vi "Main.vi"() -> ()   [LabVIEW 2015]
doc: "This template is for the Queued Message Handler design pattern.\n\nThe Event Handling Loop generates messages based on user interface actions.\n\nThe Message Handling Loop processes messages generated by the Event Handling Loop, or by other messages. The messages are string values, so new messages can be added easily to the Message Cases case structure in the Message Handling Loop. Each message cluster can also provide an optional value for Message Data, which is a variant that can be converted to whatever message-specific data is required."
uses:
  controls/Instruments.ctl
  controls/UI Data.ctl
  controls/UI Config.ctl
  Classes/Calibrator.lvclass
  Classes/34410A.lvclass
  Classes/34401A.lvclass
  Classes/8846A.lvclass
  Classes/8845A.lvclass
  Classes/U1252.lvclass
  Classes/U1213A.lvclass
  Classes/189.lvclass
  Classes/289/289.lvclass
  Classes/TY720.lvclass
  Classes/Multimeter.lvclass
  controls/Ini File Output.ctl
  support/Message Queue/Enqueue Message (Single).vi
  <vilib>/Utility/config.llb/Read Key (String).vi
  support/Developer VIs/Write Cell.vi
  support/Developer VIs/Write Cell String.vi
  <vilib>/Utility/error.llb/Error Cluster From Error Code.vi
  <vilib>/Utility/NIReport.llb/NI_report.lvclass
  <vilib>/ErrorRing/Error Ring.xnode
  support/Message Queue/Message Queue.lvlib
  support/User Event - Stop/User Event - Stop.lvlib
  <vilib>/Utility/config.llb/NI_LVConfig.lvlib
  <vilib>/addons/_office/NI_ReportGenerationToolkit.lvlib
panel:
  out "Conexão com Padrão":bool
  in  "Frequência":bool=TRUE
  in  "Bobina":enum16{"50", "75"}(ring)
  in  "Capacitância":bool=TRUE
  in  "Próxima Calibração":timestamp format="%<%x>T"
  in  "Multimetro":T1
  in  "Corrente AC":bool=TRUE
  in  "Corrente DC":bool=TRUE
  in  "Parar":bool
  in  "Número de Controle":string
  in  "Patrimônio":string
  in  "Tipo de Calibração":enum32{"Nova", "Recalibração"}(radio)
  in  "Tensão DC":bool=TRUE
  in  "Tensão AC":bool=TRUE
  in  "Resistência":bool=TRUE
  in  "Finalizar Aplicativo":bool
  in  "Iniciar Calibração":bool
  # "CALIBRAÇÃO AUTOMÁTICA\nDE MULTÍMETROS DIGITAIS"
  # "Selecione as Grandezas\nElétricas"
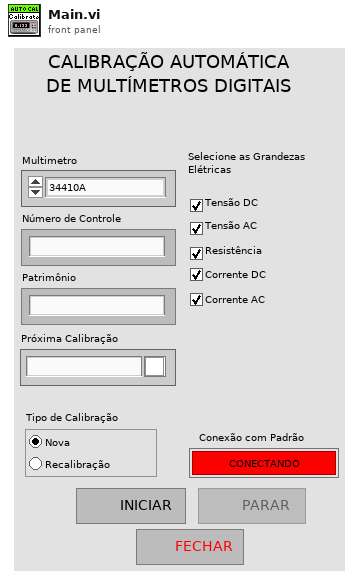
[diagram p1: front panel]
types:
  T1 = typedef "Instruments.ctl" = enum16{"34410A", "34401A", "U1252B", "U1252A", "U1213A", "8845A", "8846A", "189", "289", "DMM4050", "TY720"}
  T2 = typedef "UI Data.ctl" = cluster{"Voltage DC":refnum<vi>, "Voltage AC":refnum<vi>, "Resistance":refnum<vi>, "Current DC":refnum<vi>, "Current AC":refnum<vi>, "Finalizar":refnum<vi>, "Iniciar Cal":refnum<vi>, "Stop":refnum<vi>, "Conexão com Padrão":refnum<vi>, "Número de Controle":refnum<vi>, "Patrimônio":refnum<vi>, "Próxima Calibração":refnum<vi>, "Tipo de Calibração":refnum<vi>, "Bobina":refnum<vi>, "Capacitância":refnum<vi>, "Frequência":refnum<vi>, "Bobina":refnum<vi>, "Multimetro":refnum<vi>}
  T3 = typedef "Message Queue.lvlib/All Message Queues.ctl" = cluster{"UI":refnum<queue>}
  T4 = typedef "UI Config.ctl" = enum16{"Initial Config", "Calibration Config"}
  T5 = enum16{"Standard Report", "HTML", "Word", "Excel"}
  T6 = enum16{"maximized", "minimized", "normal", "no change"}
  T7 = typedef "NI_LVConfig.lvlib/Config Data RefNum.ctl" = refnum<k1>
  T8 = typedef "Ini File Output.ctl" = cluster{"Grandeza":string, "Cel Inicio":string, "Cel Fim":string, "Frequencia":dbl, "Delay":dbl, "Valor":dbl, "Num Medições":i32, "Cel Write":string, "Multiplicador":dbl, "Message":string, "Escala":dbl, "Reset":bool}
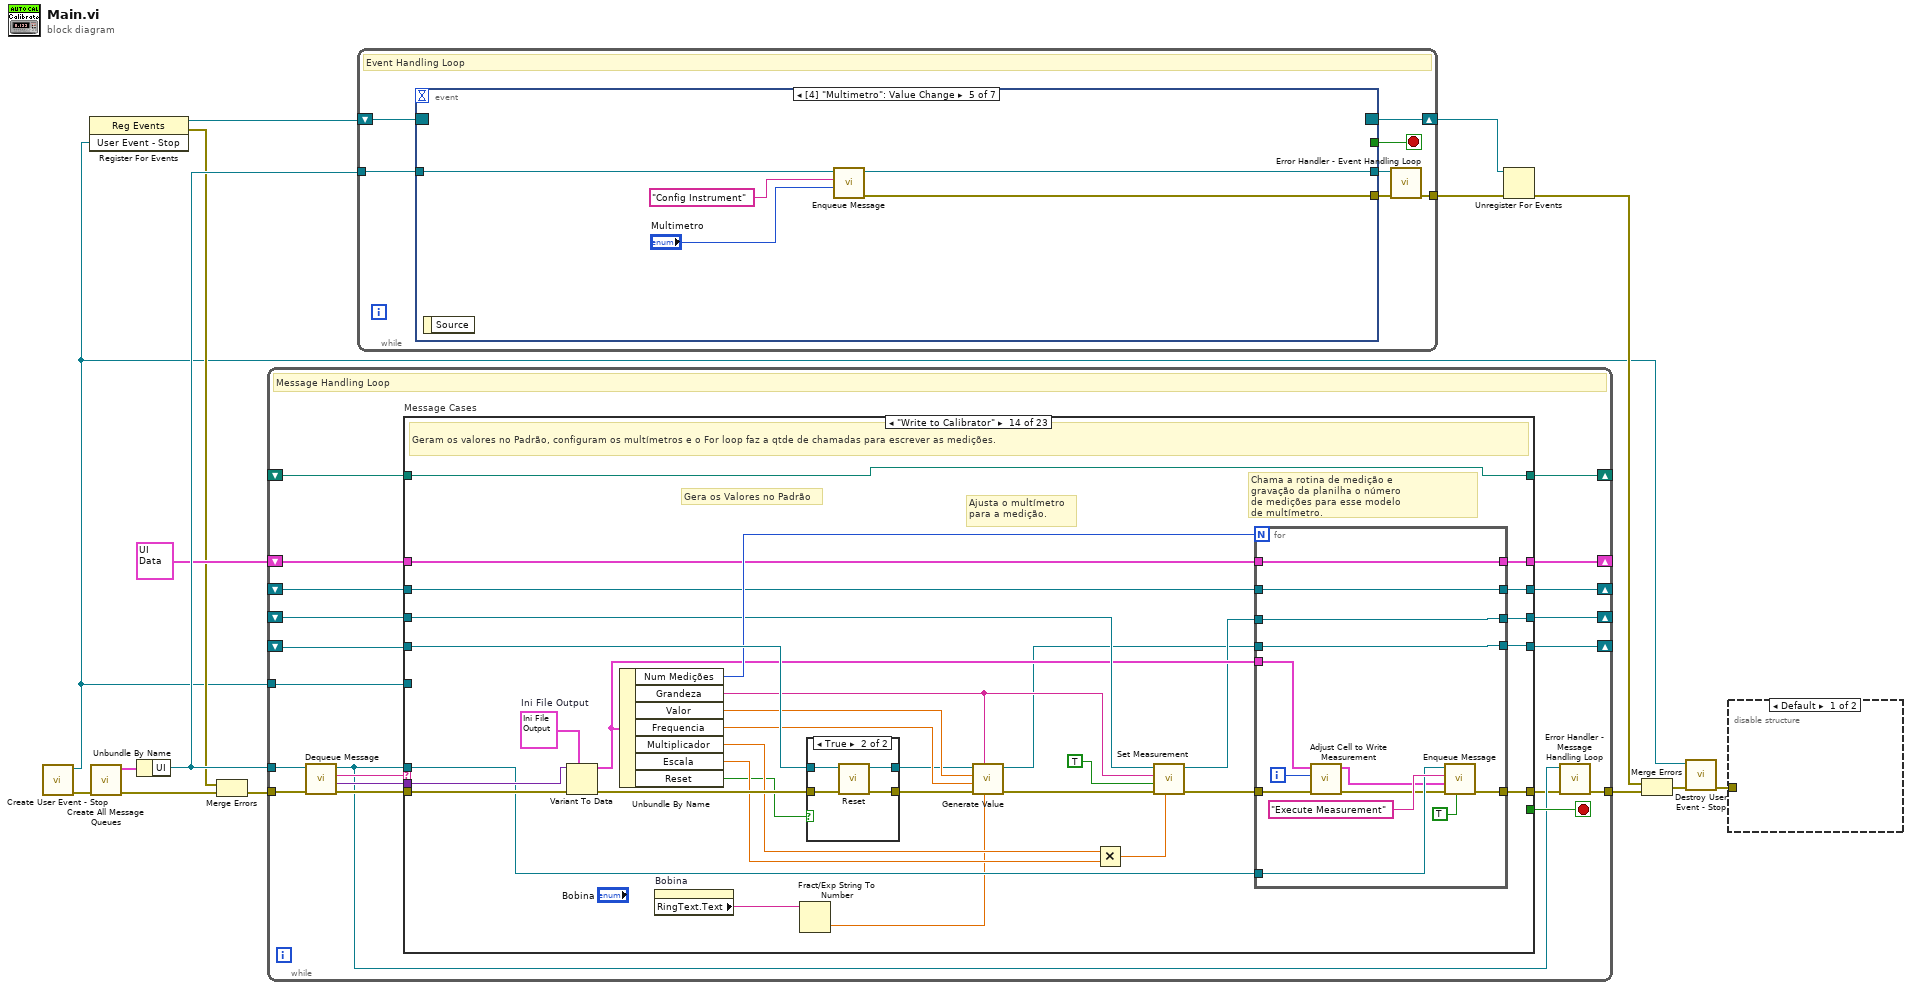
[diagram p0: block diagram]
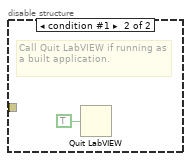
[diagram p2: hidden frame]
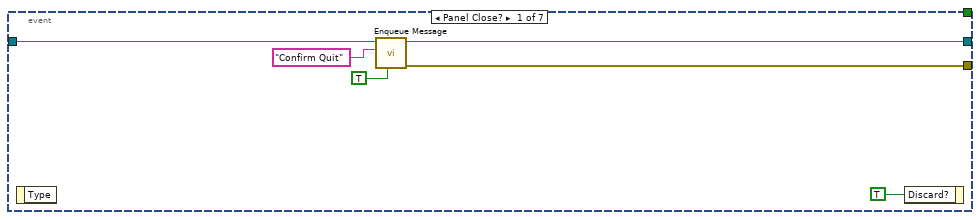
[diagram p3: hidden frame]
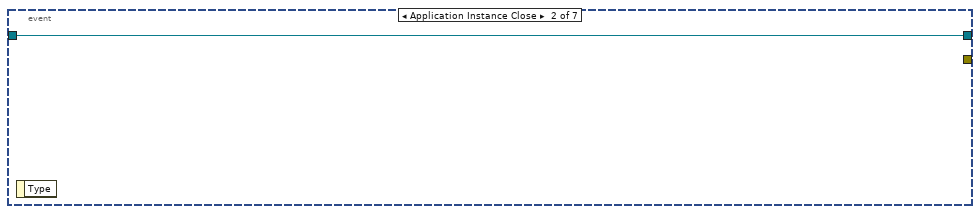
[diagram p4: hidden frame]
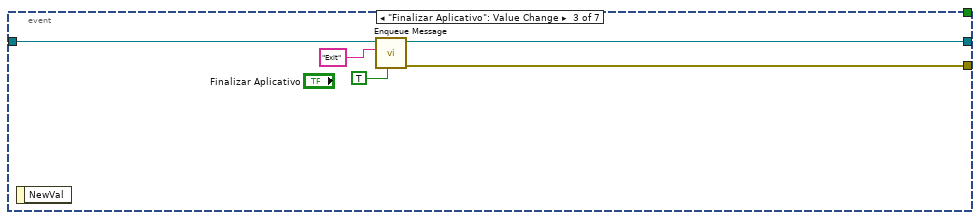
[diagram p5: hidden frame]
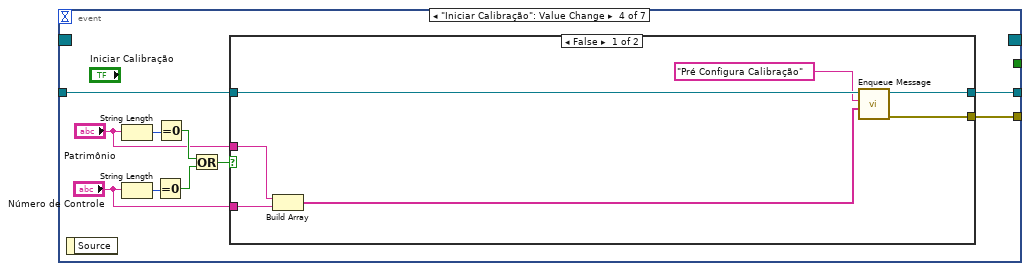
[diagram p6: hidden frame]
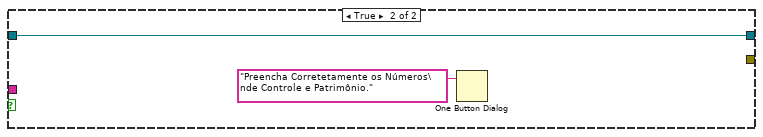
[diagram p7: hidden frame]
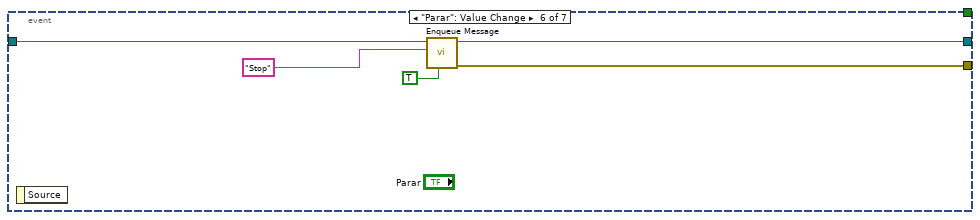
[diagram p8: hidden frame]
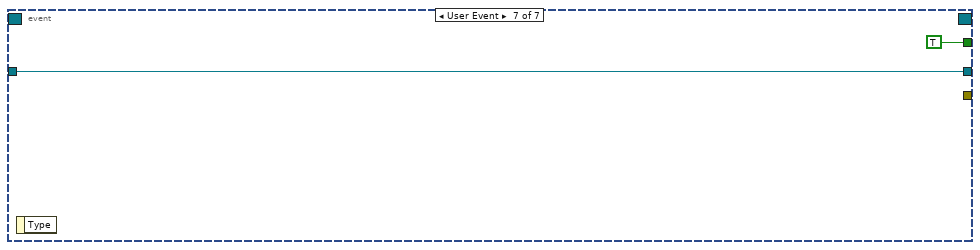
[diagram p9: hidden frame]
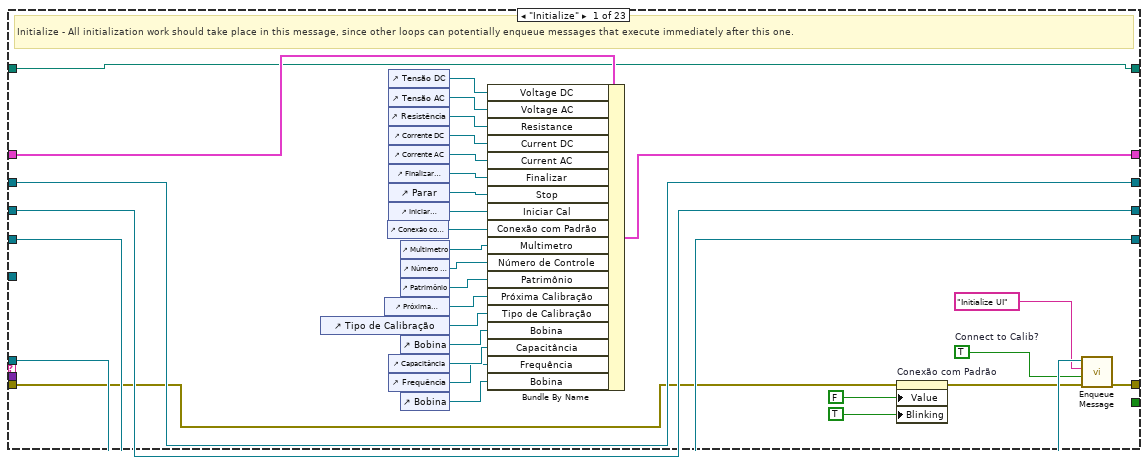
[diagram p10: hidden frame]
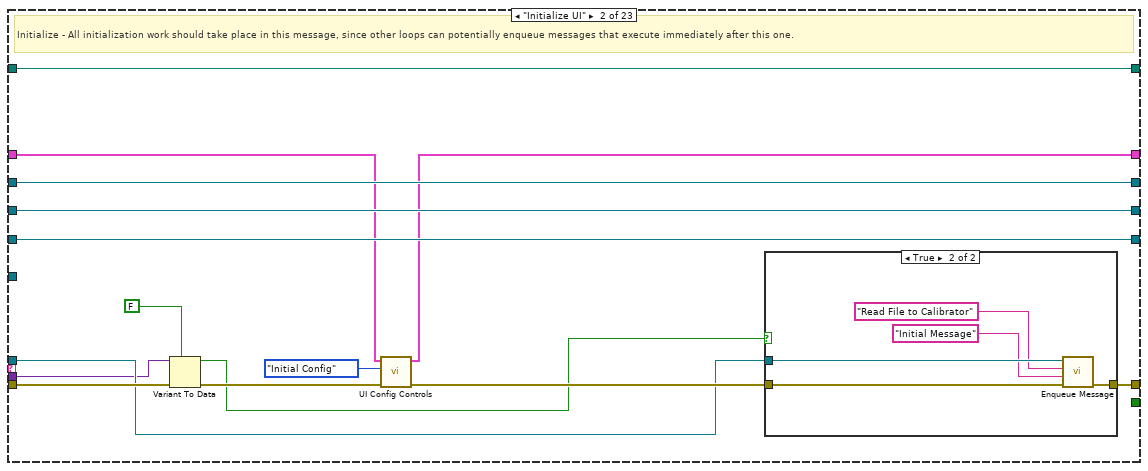
[diagram p11: hidden frame]
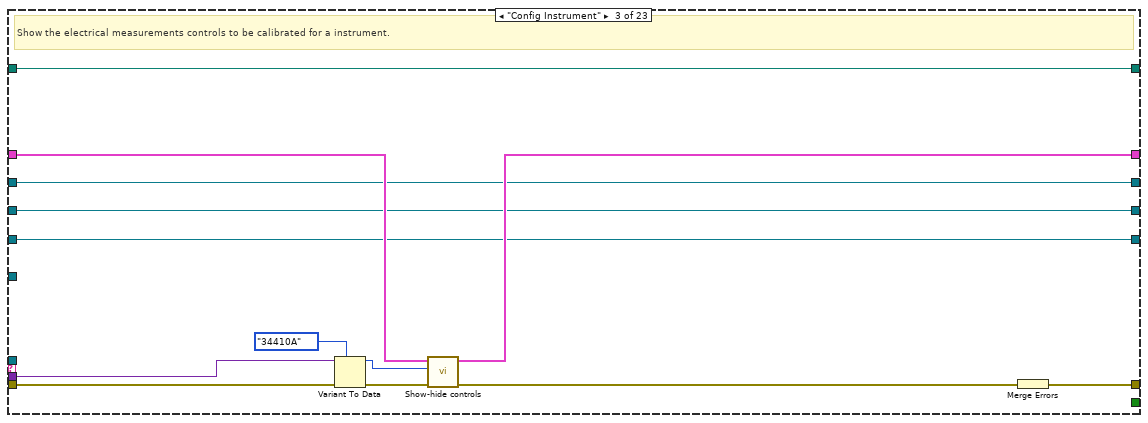
[diagram p13: hidden frame]
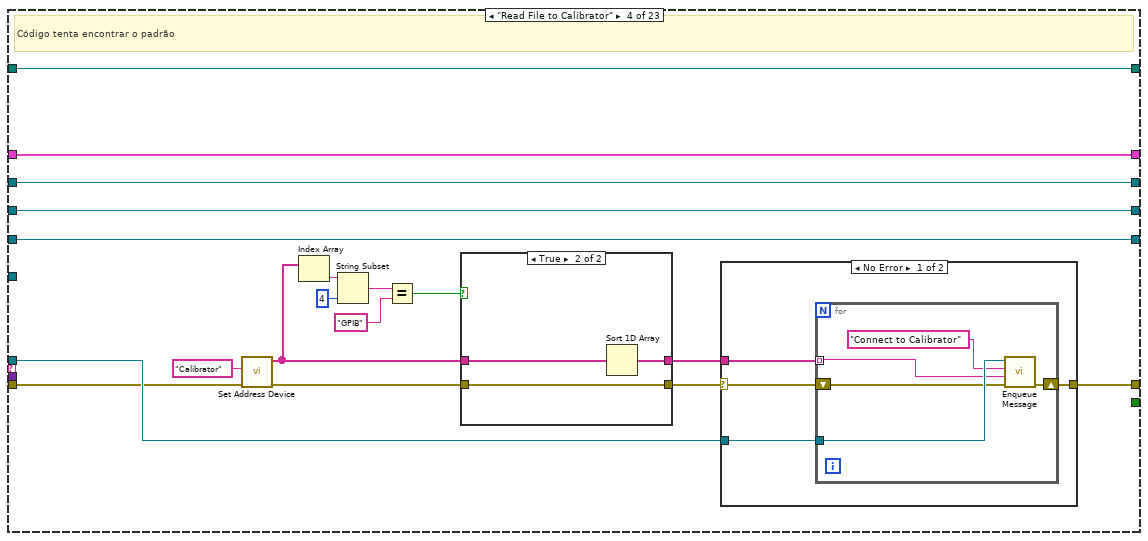
[diagram p14: hidden frame]
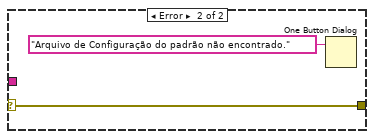
[diagram p16: hidden frame]
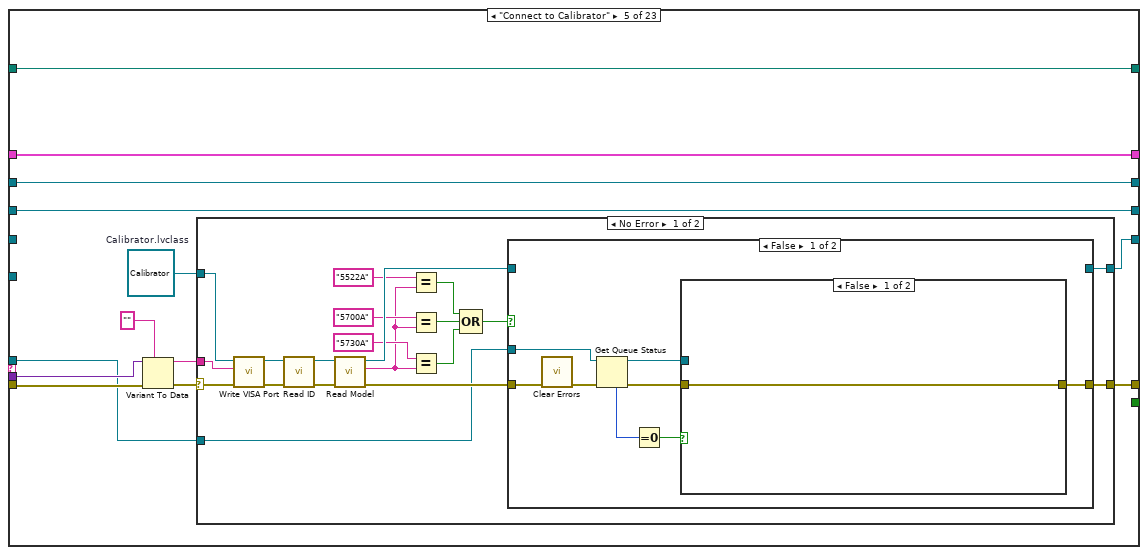
[diagram p17: hidden frame]
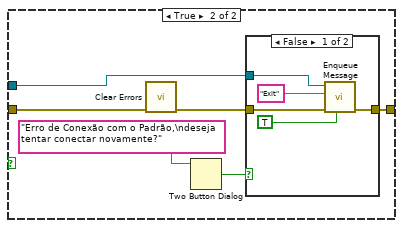
[diagram p18: hidden frame]
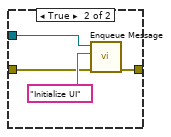
[diagram p19: hidden frame]
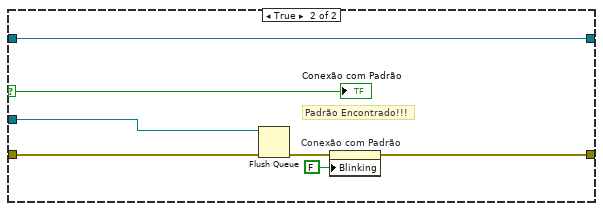
[diagram p20: hidden frame]
diagram:
  n1 = call "Create User Event - Stop.vi"() -> ("error out"=w11:errorcluster, "User Event - Stop"=w1:refnum<user-event>)  [unwired: 10 in]
  n2 = register-events(w1) -> (reference out=w4:refnum<event-registration>, error out=w2:errorcluster)  [unwired: 2 in]
  n3 = call "Create All Message Queues.vi"("error in (no error)"=w11) -> ("error out"=w15:errorcluster, "Message Queues out"=w14:T3)  [unwired: 9 in]
  n4 = Unbundle By Name(w14) -> ("UI"=w12:refnum<queue>)
  n5 = Merge Errors(w2, w15) -> (w3:errorcluster)
  n6 = while {
    tunnel: w12 -> [w27]
    shift-right: [w34] -> _
    shift-left: T2 {"Voltage DC"=refnum, "Voltage AC"=refnum, "Resistance"=refnum, "Current DC"=refnum, "Current AC"=refnum, "Finalizar"=refnum, "Iniciar Cal"=refnum, "Stop"=refnum, "Conexão com Padrão"=refnum, "Número de Controle"=refnum, "Patrimônio"=refnum, "Próxima Calibração"=refnum, "Tipo de Calibração"=refnum, "Bobina"=refnum, "Capacitância"=refnum, "Frequência"=refnum, "Bobina"=refnum, "Multimetro"=refnum} ("Data Cluster") -> [w35]
    tunnel: w1 -> [w32]
    tunnel: w3 -> [w31]
    tunnel: [w25] -> w13
    shift-right: [w18] -> _
    shift-left: _ -> [w23]
    shift-right: [w22] -> _
    shift-left: _ -> [w21]
    shift-right: [w20] -> _
    shift-left: _ -> [w19]
    shift-right: [w17] -> _
    shift-left: _ -> [w16]
    stop <- w33 stop-if-true
    # "Message Handling Loop"
    n7 = call "Dequeue Message.vi"("error in (no error)"=w31, "Message Queue"=w27) -> ("error out"=w30:errorcluster, "Message Data"=w28:variant, "Message"=w29:string, "dup Message Queue"=w26:refnum<queue>)  [unwired: 6 in]
    n8 = case "Message Cases" shown="\"Write to Calibrator\"" w29 {
      selector: w29 -> [_ _ _ _ _ _ _ _ _ _ _ _ _ _ _ _ _ _ _ _ _ _ w892]
      tunnel: w26 -> [w66 w73 _ w117 w138 w204 w246 w283 w356 _ w480 w529 _ w675 w718 w747 _ w841 w850 _ _ w887 _]
      tunnel: w30 -> [w40 w78 w98 w114 w143 w210 w245 w292 w352 w464 w490 w546 w618 w684 w728 w753 w806 w840 w854 w861 w868 w882 _]
      tunnel: [w67 w82 w101 w118 w136 w205 w241 w284 w339 w443 w476 w539 w614 w674 w714 w744 w800 w809 w852 w859 w867 w885 w893] -> w24
      tunnel: w35 -> [w65 w77 w95 w119 w148 w214 w240 w291 w363 w468 w492 w545 w605 w656 w729 w737 w805 w808 w853 w860 w866 w878 w894]
      tunnel: [w59 w76 w93 w119 w148 w214 w239 w291 w363 w468 w492 w545 w606 w655 w729 w736 w805 w807 w853 w860 w866 w876 w894] -> w34
      tunnel: [_ _ _ _ _ _ _ _ _ _ _ _ _ _ _ _ _ _ _ _ _ TRUE _] -> w33
      tunnel: w28 -> [_ w69 w100 _ w141 _ w244 w290 w351 w463 w489 w538 w613 w683 w727 w752 w804 _ _ _ _ w879 _]
      tunnel: w32 -> [_ _ _ _ _ _ _ _ _ _ _ _ _ _ _ _ _ _ _ _ _ w884 _]
      tunnel: [w53 w81 w92 w112 w137 w207 w258 w282 w362 w467 w491 w534 w609 w658 w723 w739 w799 w813 w847 w858 w865 w871 w891] -> w18
      tunnel: w23 -> [w53 w81 w92 w112 _ w208 w258 w289 w362 w467 w491 w535 w610 w680 w723 w740 w799 w815 w847 w858 w865 w872 w891]
      tunnel: [w56 w80 w91 w116 w147 w213 w257 w280 w342 w466 w472 w543 w616 w662 w721 w745 w798 w818 w846 w857 w864 w875 w890] -> w22
      tunnel: w21 -> [w56 w80 w91 w116 w147 w213 w257 _ w343 w466 w473 w544 w617 w671 w722 w746 w798 w818 w846 w857 w864 w875 w890]
      tunnel: [w46 w79 w90 w115 w146 w212 w256 w276 w346 w459 w482 w537 w612 w660 w712 w750 w797 w820 w845 w856 w863 w874 w889] -> w20
      tunnel: w19 -> [w46 w79 w90 w115 w146 w212 w256 w276 w346 w459 w482 w536 w611 w661 w724 _ w797 w834 w845 w856 w863 w874 w889]
      tunnel: [w42 w72 w89 w113 w145 w201 w230 w272 w338 w441 w469 w528 w604 w654 w704 w735 w796 w819 w844 w855 w862 w869 w888] -> w17
      tunnel: w16 -> [w42 w72 w89 w113 w145 w201 w230 w272 w338 w441 w469 w528 w604 w654 w704 _ w796 w819 w844 w855 w862 w869 w888]
      frame "Initialize" {
        w41 = TRUE  # Connect to Calib?
        # "Initialize - All initialization work should take place in this message, since other loops can potentially enqueue messages that execute immediately after this one."
        n9 = control-ref of="Tipo de Calibração"() -> (w51:refnum<vi>)
        n10 = control-ref of="Próxima Calibração"() -> (w50:refnum<vi>)
        n11 = control-ref of="Conexão com Padrão"() -> (w39:refnum<vi>)
        n12 = control-ref of="Tensão DC"() -> (w64:refnum<vi>)
        n13 = control-ref of="Tensão AC"() -> (w63:refnum<vi>)
        n14 = control-ref of="Resistência"() -> (w62:refnum<vi>)
        n15 = control-ref of="Corrente DC"() -> (w61:refnum<vi>)
        n16 = control-ref of="Corrente AC"() -> (w60:refnum<vi>)
        n17 = control-ref of="Finalizar Aplicativo"() -> (w58:refnum<vi>)
        n18 = control-ref of="Parar"() -> (w55:refnum<vi>)
        n19 = control-ref of="Iniciar Calibração"() -> (w57:refnum<vi>)
        n20 = control-ref of="Capacitância"() -> (w47:refnum<vi>)
        n21 = control-ref of="Frequência"() -> (w45:refnum<vi>)
        n22 = control-ref of="Multimetro"() -> (w43:refnum<vi>)
        n23 = control-ref of="Número de Controle"() -> (w48:refnum<vi>)
        n24 = control-ref of="Patrimônio"() -> (w49:refnum<vi>)
        n25 = control-ref of="Bobina"() -> (w52:refnum<vi>)
        n26 = control-ref of="Bobina"() -> (w44:refnum<vi>)
        n27 = Bundle By Name(cluster=w65, "Voltage DC"=w64, "Voltage AC"=w63, "Resistance"=w62, "Current DC"=w61, "Current AC"=w60, "Finalizar"=w58, "Stop"=w55, "Iniciar Cal"=w57, "Conexão com Padrão"=w39, "Multimetro"=w43, "Número de Controle"=w48, "Patrimônio"=w49, "Próxima Calibração"=w50, "Tipo de Calibração"=w51, "Bobina"=w52, "Capacitância"=w47, "Frequência"=w45, "Bobina"=w44) -> (w59:T2)
        n28 = property on="Conexão com Padrão" class="Bool (strict)"(error in=w40, "Value"=FALSE ("Blinking"), "Blinking"=TRUE) -> (error out=w38:errorcluster)  [unwired: 1 in, 1 out]
        n29 = call-poly "Enqueue Message.vi"("error in (no error)"=w38, "Message Data"=w41, "Message"="Initialize UI", "Message Queue"=w66) -> ("error out"=w67:errorcluster)  [unwired: 6 in, 1 out]
      }
      frame "Initialize UI" {
        # "Initialize - All initialization work should take place in this message, since other loops can potentially enqueue messages that execute immediately after this one."
        n30 = Variant To Data(error in=w78, type=FALSE, Variant=w69) -> (data=w68:bool, error out=w71:errorcluster)
        n31 = call "UI Config Controls.vi"("Error In"=w71, "UI Configuration"=UI_Config."Initial Config", "UI Data"=w77) -> ("Error Out"=w74:errorcluster, "UI Data 2"=w76:T2)  [unwired: 7 in]
        n32 = case shown="True" w68 {
          tunnel: [w83 w88] -> w82
          tunnel: w74 -> [w83 w87]
          tunnel: w73 -> [_ w86]
          frame False {
          }
          frame True {
            n33 = call-poly "Enqueue Message.vi"("error in (no error)"=w87, "Message Data"="Initial Message" ("Initial Message"), "Message"="Read File to Calibrator", "Message Queue"=w86) -> ("error out"=w88:errorcluster)  [unwired: 6 in, 1 out]
          }
        }
      }
      frame "Config Instrument" {
        # "Show the electrical measurements controls to be calibrated for a instrument."
        n34 = Variant To Data(error in=w98, type=Instruments."34410A" ("Multimetro"), Variant=w100) -> (data=w96:T1, error out=w97:errorcluster)
        n35 = call "Show-hide controls.vi"("Error In"=w97, "Multimetro"=w96, "Data In"=w95) -> ("Error Out"=w94:errorcluster, "Data Out"=w93:T2)  [unwired: 7 in]
        n36 = Merge Errors(w94) -> (w101:errorcluster)
      }
      frame "Read File to Calibrator" {
        # "Código tenta encontrar o padrão"
        n37 = call "Set Address Device.vi"("error in (no error)"=w114, "Device"="Calibrator") -> ("error out"=w103:errorcluster, "find list"=w104:string[])  [unwired: 8 in]
        n38 = Index Array(array=w104) -> (element=w109:string)  [unwired: 1 in]
        n39 = String Subset(string=w109, length (rest)=4 ("length (rest)")) -> (substring=w106:string)  [unwired: 1 in]
        n40 = Equal?(x=w106, y="GPIB") -> (x = y?=w107:bool)
        n41 = case shown="True" w107 {
          tunnel: [w120 w124] -> w111
          tunnel: w104 -> [w120 w123]
          tunnel: w103 -> [w121 w122]
          tunnel: [w121 w122] -> w102
          frame False {
          }
          frame True {
            n42 = Sort 1D Array(array=w123) -> (sorted array=w124:string[])
          }
        }
        n43 = case shown="No Error" w102 {
          selector: w102 -> [w126 w135]
          tunnel: [w128 w135] -> w118
          tunnel: w117 -> [w127 _]
          tunnel: w111 -> [w125 _]
          frame No Error {
            n44 = for {
              tunnel: w127 -> [w132]
              shift-right: [w133] -> w128
              shift-left: w126 -> [w131]
              tunnel: w125 -> [w130] mode=indexing
              n45 = call-poly "Enqueue Message.vi"("error in (no error)"=w131, "Message Data"=w130, "Message"="Connect to Calibrator", "Message Queue"=w132) -> ("error out"=w133:errorcluster)  [unwired: 6 in, 1 out]
            }
          }
          frame Error {
            n46 = One Button Dialog(message="Arquivo de Configuração do padrão não encontrado.") -> ()  [unwired: 1 in, 1 out]
          }
        }
      }
      frame "Connect to Calibrator" {
        w144 = refnum<class "Calibrator.lvclass"> refnum  # Calibrator.lvclass
        n47 = Variant To Data(error in=w143, type="", Variant=w141) -> (data=w140:string, error out=w139:errorcluster)
        n48 = case shown="No Error" w139 {
          selector: w139 -> [w160 w200]
          tunnel: w144 -> [w168 _]
          tunnel: [w165 w200] -> w136
          tunnel: w138 -> [w164 _]
          tunnel: [w163 _] -> w137
          tunnel: w140 -> [w161 _]
          frame No Error {
            n49 = call-dynamic "Write VISA Port.vi"("error in (no error)"=w160, "VISA Port"=w161, "Device in"=w168) -> ("error out"=w158:errorcluster, "Device out"=w159:refnum<class "Calibrator.lvclass">)  [unwired: 7 in]
            n50 = call-dynamic "Read ID.vi"("error in (no error)"=w158, "Calibrator in"=w159) -> ("error out"=w156:errorcluster, "Calibrator out"=w157:refnum<class "Calibrator.lvclass">)  [unwired: 8 in]
            n51 = call-dynamic "Read Model.vi"("error in (no error)"=w156, "Device in"=w157) -> ("error out"=w166:errorcluster, "Model"=w153:string, "Device out"=w162:refnum<class "Calibrator.lvclass">)  [unwired: 7 in]
            n52 = Equal?(x="5522A", y=w153) -> (x = y?=w151:bool)
            n53 = Equal?(x="5700A", y=w153) -> (x = y?=w150:bool)
            n54 = Equal?(x="5730A", y=w153) -> (x = y?=w149:bool)
            n55 = Compound Arithmetic op=OR(w151, w150, w149) -> (w167:bool)
            n56 = case shown="False" w167 {
              selector: w167 -> [_ w198]
              tunnel: w166 -> [w171 w194]
              tunnel: [w176 w197] -> w165
              tunnel: w164 -> [w175 w195]
              tunnel: [_ w196] -> w163
              tunnel: w162 -> [_ w196]
              frame False {
                n57 = call <vilib>:"Clear Errors.vi"("error in (no error)"=w171) -> ("error out"=w170:errorcluster)  [unwired: 5 in, 1 out]
                n58 = Get Queue Status(queue=w175, error in (no error)=w170) -> (queue out=w172:refnum<queue>, error out=w173:errorcluster, # elements in queue=w169:i32)  [unwired: 1 in, 5 out]
                n59 = Equal To 0?(x=w169) -> (x = 0?=w174:bool)
                n60 = case shown="False" w174 {
                  tunnel: [w177 w181] -> w176
                  tunnel: w172 -> [_ w180]
                  tunnel: w173 -> [w177 w179]
                  frame False {
                  }
                  frame True {
                    n61 = call <vilib>:"Clear Errors.vi"("error in (no error)"=w179) -> ("error out"=w178:errorcluster)  [unwired: 5 in, 1 out]
                    n62 = Two Button Dialog(message="Erro de Conexão com o Padrão,\ndeseja tentar conectar novamente?") -> (T button?=w182:bool)  [unwired: 2 in]
                    n63 = case shown="False" w182 {
                      tunnel: w178 -> [w186 w189]
                      tunnel: [w185 w191] -> w181
                      tunnel: w180 -> [w184 w190]
                      frame False {
                        n64 = call-poly "Enqueue Message.vi"("Priority Message? (F)"=TRUE, "error in (no error)"=w186, "Message"="Exit", "Message Queue"=w184) -> ("error out"=w185:errorcluster)  [unwired: 6 in, 1 out]
                      }
                      frame True {
                        n65 = call-poly "Enqueue Message.vi"("error in (no error)"=w189, "Message"="Initialize UI", "Message Queue"=w190) -> ("error out"=w191:errorcluster)  [unwired: 7 in, 1 out]
                      }
                    }
                  }
                }
              }
              frame True {
                # "Padrão Encontrado!!!"
                n66 = Flush Queue(queue=w195, error in (no error)=w194) -> (error out=w193:errorcluster)  [unwired: 2 out]
                n67 = property on="Conexão com Padrão" class="Bool (strict)"(error in=w193, "Blinking"=FALSE) -> (error out=w197:errorcluster)  [unwired: 1 in, 1 out]
                "Conexão com Padrão" <- w198
              }
            }
          }
          frame Error {
          }
        }
      }
      frame "Checa Padrão" {
        n68 = call "FGV Config File.vi"("Error In"=w210, "Set/Get"=enum16{"Get", "Set"}."Get") -> ("Error Out"=w209:errorcluster, "Padrão Out"=w202:string[])  [unwired: 7 in, 1 out]
        n69 = for {
          tunnel: w209 -> [w229]
          tunnel: w208 -> [w228]
          tunnel: [w227] -> w207
          tunnel: [w226] -> w203
          tunnel: [w224] -> w206
          tunnel: w202 -> [w223] mode=indexing
          stop <- w224 stop-if-true
          n70 = call-dynamic "Read Model.vi"("error in (no error)"=w229, "Device in"=w228) -> ("error out"=w226:errorcluster, "Model"=w225:string, "Device out"=w227:refnum<class "Calibrator.lvclass">)  [unwired: 7 in]
          n71 = Equal?(x=w225, y=w223) -> (x = y?=w224:bool)
        }
        n72 = case shown="False" w206 {
          tunnel: [w215 w222] -> w205
          tunnel: w204 -> [w220 _]
          tunnel: w203 -> [w219 w222]
          frame False {
            n73 = Flush Queue(queue=w220, error in (no error)=w219) -> (queue out=w217:refnum<queue>, error out=w216:errorcluster)  [unwired: 1 out]
            n74 = call-poly "Enqueue Message.vi"("error in (no error)"=w216, "Message"="Initialize UI", "Message Queue"=w217) -> ("error out"=w215:errorcluster)  [unwired: 7 in, 1 out]
            n75 = One Button Dialog(message="O padrão conectado não pode ser utilizado\npara calibrar esse instrumento.") -> ()  [unwired: 1 in, 1 out]
          }
          frame True {
          }
        }
      }
      frame "Pré Configura Calibração" {
        n76 = Variant To Data(error in=w245, type=string[] [], Variant=w244) -> (data=w242:string[], error out=w237:errorcluster)
        n77 = call "UI Config Controls.vi"("Error In"=w237, "UI Configuration"=UI_Config."Calibration Config", "UI Data"=w240) -> ("Error Out"=w236:errorcluster, "UI Data 2"=w239:T2)  [unwired: 7 in]
        n78 = local read "Multimetro"() -> (w253:T1)
        n79 = case shown="\"8846A\"" w253 {
          tunnel: [w259 w260 w261 w262 w263 w264 w265 w266 w267] -> w254
          frame "34410A", Default {
            w259 = refnum<class "34410A.lvclass"> refnum  # 34410A.lvclass
          }
          frame "34401A" {
            w260 = refnum<class "34401A.lvclass"> refnum  # 34401A.lvclass
          }
          frame "8846A" {
            w261 = refnum<class "8846A.lvclass"> refnum  # 8846A.lvclass
          }
          frame "8845A" {
            w262 = refnum<class "8845A.lvclass"> refnum  # 8845A.lvclass
          }
          frame "U1252B", "U1252A" {
            w263 = refnum<class "U1252.lvclass"> refnum  # U1252.lvclass
          }
          frame "U1213A" {
            w264 = refnum<class "U1213A.lvclass"> refnum  # U1213A.lvclass
          }
          frame "189" {
            w265 = refnum<class "189.lvclass"> refnum  # 189.lvclass
          }
          frame "289" {
            w266 = refnum<class "289.lvclass"> refnum  # 289.lvclass
          }
          frame "TY720" {
            w267 = refnum<class "TY720.lvclass"> refnum  # TY720.lvclass
          }
        }
        n80 = call-poly "Enqueue Message.vi"("error in (no error)"=w236, "Message Data"=w254, "Message"="Iniciar Calibração", "Message Queue"=w246) -> ("error out"=w247:errorcluster, "dup Message Queue"=w251:refnum<queue>)  [unwired: 6 in]
        n81 = property on="Multimetro" class="Enum (strict)"(error in=w247) -> (error out=w250:errorcluster, "RingText.Text"=w255:string)  [unwired: 1 in, 1 out]
        n82 = call-poly "Enqueue Message.vi"("error in (no error)"=w250, "Message Data"=w255, "Message"="Read General Config File", "Message Queue"=w251) -> ("error out"=w233:errorcluster, "dup Message Queue"=w234:refnum<queue>)  [unwired: 6 in]
        n83 = call-poly "Enqueue Message.vi"("error in (no error)"=w233, "Message"="Checa Padrão", "Message Queue"=w234) -> ("error out"=w232:errorcluster, "dup Message Queue"=w231:refnum<queue>)  [unwired: 7 in]
        n84 = call-poly "Enqueue Message.vi"("error in (no error)"=w232, "Message Data"=w242, "Message"="Open Excel File", "Message Queue"=w231) -> ("error out"=w241:errorcluster)  [unwired: 6 in, 1 out]
      }
      frame "Iniciar Calibração" {
        w277 = refnum<class "Multimeter.lvclass"> refnum  # Multimeter.lvclass
        # "Tenta estabelecer comunicação com o multímetro selecionado."
        n85 = property on="Multimetro" class="Enum (strict)"() -> ("RingText.Text"=w271:string)  [unwired: 2 in, 2 out]
        n86 = Variant To Data(error in=w292, type=w277, Variant=w290) -> (data=w286:refnum<class "Multimeter.lvclass">, error out=w275:errorcluster)
        n87 = local read "Multimetro"() -> (w268:T1)
        n88 = call-dynamic "Read VISA Port.vi"("Device in"=w289) -> ("VISA Port"=w288:refnum<visa-resource-name>, "Device out"=w282:refnum<class "Calibrator.lvclass">)  [unwired: 8 in, 1 out]
        n89 = call "Set Address Device.vi"("error in (no error)"=w275, "Device"=w271) -> ("error out"=w274:errorcluster, "find list"=w273:string[])  [unwired: 8 in]
        n90 = Search 1D Array(1D array=w273, element=w288) -> (index of element=w287:i32)  [unwired: 1 in]
        n91 = Delete From Array(array=w273, index=w287) -> (array with subset deleted=w270:string[])  [unwired: 1 in, 1 out]
        n92 = call "Find Port.vi"("Multimetro"=w268, "Ports Found"=w270) -> ("Addr Ports"=w269:string[])  [unwired: 9 in]
        n93 = for {
          tunnel: w274 -> [w336]
          tunnel: w286 -> [w335]
          tunnel: [w330] -> w281
          tunnel: [w329] -> w285
          tunnel: [w327] -> w279
          tunnel: [w326] -> w278
          tunnel: w269 -> [w325] mode=indexing
          stop <- w327 stop-if-true
          n94 = call-dynamic "Write VISA Port.vi"("error in (no error)"=w336, "VISA Port"=w325, "Device in"=w335) -> ("error out"=w334:errorcluster, "Device out"=w333:refnum<class "Multimeter.lvclass">)  [unwired: 7 in]
          n95 = property on="Multimetro" class="Enum (strict)"() -> ("RingText.Text"=w328:string)  [unwired: 2 in, 2 out]
          n96 = call-dynamic "Read ID.vi"("error in (no error)"=w334, "Multimeter in"=w333) -> ("error out"=w332:errorcluster, "Multimeter out"=w331:refnum<class "Multimeter.lvclass">)  [unwired: 8 in]
          n97 = call-dynamic "Read Model.vi"("error in (no error)"=w332, "Device in"=w331) -> ("error out"=w329:errorcluster, "Model"=w326:string, "Device out"=w330:refnum<class "Multimeter.lvclass">)  [unwired: 7 in]
          n98 = Equal?(x=w328, y=w326) -> (x = y?=w327:bool)
        }
        n99 = case shown="False" w279 {
          tunnel: w285 -> [w294 w314]
          tunnel: [w296 w313] -> w284
          tunnel: w283 -> [w295 w312]
          tunnel: w281 -> [_ w315]
          tunnel: [_ w315] -> w280
          tunnel: w278 -> [_ w311]
          frame False {
            n100 = call <vilib>:"Clear Errors.vi"("error in (no error)"=w294) -> ("error out"=w293:errorcluster)  [unwired: 5 in, 1 out]
            n101 = Two Button Dialog(message="Erro de Conexão com o Multímetro,\ndeseja tentar conectar novamente?") -> (T button?=w297:bool)  [unwired: 2 in]
            n102 = case shown="False" w297 {
              tunnel: w293 -> [w305 w307]
              tunnel: [w300 w309] -> w296
              tunnel: w295 -> [w304 w308]
              frame False {
                n103 = Flush Queue(queue=w304, error in (no error)=w305) -> (queue out=w301:refnum<queue>, error out=w302:errorcluster)  [unwired: 1 out]
                n104 = call-poly "Enqueue Message.vi"("error in (no error)"=w302, "Message Data"=FALSE, "Message"="Initialize UI", "Message Queue"=w301) -> ("error out"=w300:errorcluster)  [unwired: 6 in, 1 out]
              }
              frame True {
                n105 = call-poly "Enqueue Message.vi"("Priority Message? (F)"=TRUE, "error in (no error)"=w307, "Message"="Iniciar Calibração", "Message Queue"=w308) -> ("error out"=w309:errorcluster)  [unwired: 6 in, 1 out]
              }
            }
          }
          frame True {
            n106 = disable-structure shown="Disabled" {
              disable-tunnel: w314 -> [w322 w324]
              disable-tunnel: [w321 w324] -> w313
              disable-tunnel: w312 -> [w320 _]
              disable-tunnel: w311 -> [w318 _]
              frame Disabled {
                # "Multímetro Encontrado"
                n107 = Concatenate Strings("Config Files\\" ("string"), w318, ".ini" ("string")) -> (w316:string)
                n108 = call-poly "Enqueue Message.vi"("error in (no error)"=w322, "Message Data"=w316, "Message"="Read INI File", "Message Queue"=w320) -> ("error out"=w321:errorcluster)  [unwired: 6 in, 1 out]
              }
              frame Enabled {
              }
            }
          }
        }
      }
      frame "Read INI File" {
        # "Read INI file. Get Electrical parameters, Cell for read in Excel file and delay time."
        n109 = call <vilib>:"Application Directory.vi"() -> ("Application Directory"=w353:path)
        n110 = Variant To Data(error in=w352, type="", Variant=w351) -> (data=w349:string, error out=w347:errorcluster)
        n111 = Build Path(base path=w353, name or relative path=w349) -> (appended path=w348:path)
        n112 = call <vilib>:"Open Config Data.vi"("error in (no error)"=w347, "configuration file path"=w348) -> ("error out"=w361:errorcluster, "refnum"=w360:T7)  [unwired: 7 in, 1 out]
        n113 = call <vilib>:"Get Section Names.vi"("error in (no error)"=w361, "refnum"=w360) -> ("error out"=w359:errorcluster, "section names"=w358:string[], "refnum out"=w357:T7)  [unwired: 7 in]
        n114 = for {
          tunnel: w359 -> [w376]
          tunnel: w358 -> [w370] mode=indexing
          tunnel: w357 -> [w377]
          tunnel: [w385] -> w354
          tunnel: w356 -> [w379]
          tunnel: [w384] -> w355
          tunnel: [w383] -> w340
          tunnel: "Grandeza" ("key") -> [w372]
          n115 = call-poly <vilib>:"Read Key.vi"("section"=w370, "error in (no error)"=w376, "key"=w372, "refnum"=w377) -> ("error out"=w375:errorcluster, "value"=w374:string, "refnum out"=w373:T7)  [unwired: 4 in, 1 out]
          n116 = case shown="\"Tensao VDC\", \"Tensao mVDC\", Default" w374 {
            selector: w374 -> [w389 w396 w402 w408 w414 w420 w425]
            tunnel: w373 -> [w391 w397 w403 w409 w415 w421 w424]
            tunnel: [w391 w397 w403 w409 w415 w421 w424] -> w382
            tunnel: w375 -> [w390 w395 w401 w406 w413 w417 w423]
            tunnel: [w390 w395 w401 w406 w413 w417 w423] -> w381
            tunnel: [w389 w396 w402 w408 w414 w420 w425] -> _
            tunnel: [w388 w394 w400 w407 w412 w419 w426] -> w380
            tunnel: w379 -> [w388 w394 w400 w407 w412 w419 w426]
            tunnel: ["Tensão DC" "Tensão AC" "Resistência" "Capacitância" "Corrente DC" "Corrente AC" "Frequência"] -> w378
            tunnel: [w386 w392 w398 w404 w410 w416 w422] -> w371
            tunnel: w370 -> [w386 w392 w398 w404 w410 w416 w422]
            frame "Tensao VDC", "Tensao mVDC", Default {
            }
            frame "Slow 3Hz", "Tensao VAC", "Tensao VAC Filtro Ligado", "Tensao VAC LoZ", "Tensao mVAC", "Tensao mVAC Filtro Ligado" {
            }
            frame "Resistencia", "Resistencia 2W", "Resistencia 4W" {
            }
            frame "Capacitancia" {
            }
            frame "Alicate DC", "Alicate DC Ini", "Corrente DC", "Corrente mDC", "Corrente uDC" {
            }
            frame "Alicate AC", "Corrente AC", "Corrente mAC", "Corrente uAC" {
            }
            frame "Frequencia" {
            }
          }
          n117 = case shown="True" w378 {
            tunnel: w382 -> [w430 w440]
            tunnel: w381 -> [w429 w439]
            tunnel: w371 -> [_ w438]
            tunnel: [w430 w437] -> w385
            tunnel: [w429 w433] -> w384
            tunnel: w380 -> [w428 w432]
            tunnel: [w428 w431] -> w383
            frame False {
            }
            frame True {
              n118 = call "Read Ini File Instrument.vi"("error in (no error)"=w439, "Escala"=w438, "Refnum in"=w440) -> ("error out"=w436:errorcluster, "Ini Output"=w435:T8, "Refnum out"=w437:T7)  [unwired: 6 in]
              n119 = call-poly "Enqueue Message.vi"("error in (no error)"=w436, "Message Data"=w435, "Message"="Read Excel File", "Message Queue"=w432) -> ("error out"=w433:errorcluster, "dup Message Queue"=w431:refnum<queue>)  [unwired: 6 in]
            }
          }
        }
        n120 = call <vilib>:"Close Config Data.vi"("error in (no error)"=w355, "refnum"=w354) -> ("error out"=w341:errorcluster)  [unwired: 8 in, 1 out]
        n121 = call-dynamic "Read Model.vi"("error in (no error)"=w341, "Device in"=w343) -> ("error out"=w344:errorcluster, "Model"=w345:string, "Device out"=w342:refnum<class "Multimeter.lvclass">)  [unwired: 7 in]
        n122 = case shown="\"34410A\"" w345 {
          selector: w345 -> [_ w365]
          tunnel: w344 -> [w364 w368]
          tunnel: [w364 w367] -> w339
          tunnel: w340 -> [_ w366]
          frame "False", Default {
          }
          frame "34410A" {
            n123 = call-poly "Enqueue Message.vi"("error in (no error)"=w368, "Message Data"=w365, "Message"="Special Initiate", "Message Queue"=w366) -> ("error out"=w367:errorcluster)  [unwired: 6 in, 1 out]
          }
        }
      }
      frame "Read General Config File" {
        # "Read INI file. Get Electrical parameters, Cell for read in Excel file and delay time."
        n124 = call <vilib>:"Application Directory.vi"() -> ("Application Directory"=w465:path)
        n125 = Variant To Data(error in=w464, type="", Variant=w463) -> (data=w456:string, error out=w460:errorcluster)
        n126 = Build Path(base path=w465, name or relative path="Config Files\\General_Config.ini") -> (appended path=w461:path)
        n127 = call "Read General File.vi"("error in (no error)"=w460, "Session"=w456, "path"=w461) -> ("error out"=w449:errorcluster, "Controle"=w445:string, "Padrao"=w453:string, "path"=w451:path, "Patrim"=w444:string, "Data"=w446:string, "Hoje"=w442:string)  [unwired: 2 in]
        n128 = Spreadsheet String To Array(delimiter (Tab)=",", format string="", spreadsheet string=w453, array type (2D Dbl)=string[] [] ("format string")) -> (array=w450:string[])
        n129 = call "FGV Config File.vi"("Padrão"=w450, "Error In"=w449, "Standard Path"=w451, "Set/Get"=enum16{"Get", "Set"}."Set") -> ("Error Out"=w448:errorcluster)  [unwired: 5 in, 2 out]
        n130 = call "Data to Excel.vi"("Hoje"=w442, "Proxima"=w446, "Error In"=w448, "Control"=enum16{"Get", "Set"}."Set", "Patrim"=w444, "Controle"=w445) -> ("Error Out"=w443:errorcluster)  [unwired: 1 in, 4 out]
      }
      frame "Read Excel File" {
        w488 = T8 {"Grandeza"="", "Cel Inicio"="", "Cel Fim"="", "Frequencia"=0.0, "Delay"=0.0, "Valor"=0.0, "Num Medições"=0, "Cel Write"="", "Multiplicador"=0.0, "Message"="", "Escala"=0.0, "Reset"=FALSE}  # Ini File Output
        # "Read INI file. Get Electrical parameters, Cell for read in Excel file and delay time."
        n131 = Variant To Data(error in=w490, type=w488, Variant=w489) -> (data=w477:T8, error out=w481:errorcluster)
        n132 = Unbundle By Name(w477) -> ("Cel Inicio"=w487:string, "Cel Fim"=w484:string, "Grandeza"=w470:string)
        n133 = call-poly "Enqueue Message.vi"("error in (no error)"=w481, "Message Data"=w477, "Message"="Message Box", "Message Queue"=w480) -> ("error out"=w475:errorcluster, "dup Message Queue"=w479:refnum<queue>)  [unwired: 6 in]
        n134 = call <vilib>:"Excel Get Excel Location.vi"("cell's name"=w484) -> ("row"=w483:i32)  [unwired: 1 out]
        n135 = call <vilib>:"Excel Get Excel Location.vi"("cell's name"=w487) -> ("row"=w486:i32, "column"=w485:i32)
        n136 = call-dynamic "Read Model.vi"("error in (no error)"=w475, "Device in"=w473) -> ("error out"=w474:errorcluster, "Model"=w471:string, "Device out"=w472:refnum<class "Multimeter.lvclass">)  [unwired: 7 in]
        n137 = while {
          tunnel: w477 -> [w499]
          shift-right: [w502] -> _
          shift-left: w486 -> [w501]
          tunnel: w483 -> [w506]
          tunnel: w479 -> [w495]
          tunnel: [w504] -> w476
          tunnel: w485 -> [w500]
          tunnel: w482 -> [w497]
          tunnel: w474 -> [w496]
          tunnel: w471 -> [w494]
          tunnel: w470 -> [w493]
          i -> [w508]
          stop <- w507 stop-if-true
          n138 = case shown="\"True\", Default" w494 {
            tunnel: w508 -> [w515 w527]
            tunnel: [w513 w526] -> w505
            tunnel: [w512 w525] -> w502
            tunnel: w501 -> [w516 w524]
            tunnel: w500 -> [w517 w523]
            tunnel: w499 -> [w518 w522]
            tunnel: [w511 w521] -> w498
            tunnel: w497 -> [w510 w520]
            tunnel: w496 -> [w514 w519]
            tunnel: w493 -> [w509 _]
            frame "TY720" {
              n139 = call "Increment Row TY720.vi"("column"=w517, "Iteration"=w515, "row"=w516, "error in (no error)"=w514, "Grandeza"=w509, "NI_report in"=w510, "Ini File Output in"=w518) -> ("error out"=w513:errorcluster, "Last Row"=w512:i32, "Ini File Output out"=w511:T8)  [unwired: 2 in]
            }
            frame "True", Default {
              n140 = call "Increment Calibration Row.vi"("row"=w524, "Iteration"=w527, "column"=w523, "error in (no error)"=w519, "NI_report in"=w520, "Ini File Output in"=w522) -> ("error out"=w526:errorcluster, "Last Row"=w525:i32, "Ini File Output out"=w521:T8)  [unwired: 3 in]
            }
          }
          n141 = Equal?(x=w502, y=w506) -> (x = y?=w507:bool)
          n142 = call-poly "Enqueue Message.vi"("error in (no error)"=w505, "Message Data"=w498, "Message"="Write to Calibrator", "Message Queue"=w495) -> ("error out"=w504:errorcluster)  [unwired: 6 in, 1 out]
        }
      }
      frame "Message Box" {
        w533 = T8 {"Grandeza"="", "Cel Inicio"="", "Cel Fim"="", "Frequencia"=0.0, "Delay"=0.0, "Valor"=0.0, "Num Medições"=0, "Cel Write"="", "Multiplicador"=0.0, "Message"="", "Escala"=0.0, "Reset"=FALSE}  # Ini File Output
        n143 = Variant To Data(error in=w546, type=w533, Variant=w538) -> (data=w532:T8, error out=w540:errorcluster)
        n144 = Unbundle By Name(w532) -> ("Grandeza"=w530:string, "Message"=w531:string)
        n145 = String Length(string=w531) -> (length=w542:i32)
        n146 = Equal To 0?(x=w542) -> (x = 0?=w541:bool)
        n147 = case shown="False" w541 {
          tunnel: w544 -> [w558 w603]
          tunnel: [w557 w603] -> w543
          tunnel: w531 -> [w554 _]
          tunnel: w540 -> [w551 w602]
          tunnel: [w556 w602] -> w539
          tunnel: [w559 w601] -> w537
          tunnel: w536 -> [w559 w601]
          tunnel: w535 -> [w550 w600]
          tunnel: [w549 w600] -> w534
          tunnel: w530 -> [w555 _]
          tunnel: w529 -> [w552 _]
          frame False {
            n148 = call-dynamic "Reset.vi"("error in (no error)"=w551, "Calibrator in"=w550) -> ("error out"=w547:errorcluster, "Calibrator out"=w549:refnum<class "Calibrator.lvclass">)  [unwired: 8 in]
            n149 = flat-sequence {
              tunnel: w554 -> [w562]
              tunnel: [w561] -> w553
              tunnel: [w560] -> w548
              tunnel: w547 -> [w560]
              frame #0 {
                n150 = call <vilib>:"Beep.vi"() -> ()  [unwired: 12 in]
                n151 = Two Button Dialog(message=w562) -> (T button?=w561:bool)  [unwired: 2 in]
              }
            }
            n152 = while {
              tunnel: w548 -> [w571]
              tunnel: w558 -> [w570]
              tunnel: [w569] -> w557
              tunnel: [w568] -> w556
              tunnel: w555 -> [w566]
              tunnel: w554 -> [w567]
              tunnel: w553 -> [w564]
              tunnel: w552 -> [w563]
              stop <- w565 stop-if-true
              n153 = case shown="True" w564 {
                selector: w564 -> [w577 _]
                tunnel: w571 -> [w575 w588]
                tunnel: w570 -> [w578 w587]
                tunnel: [w578 w586] -> w569
                tunnel: [w576 w585] -> w568
                tunnel: w567 -> [_ w583]
                tunnel: w566 -> [_ w581]
                tunnel: [w572 w580] -> w565
                tunnel: w563 -> [w574 w579]
                frame False {
                  n154 = Not(x=w577) -> (.not. x?=w573:bool)
                  n155 = call "Cancel Calibration.vi"("error in (no error)"=w575, "Boolean"=w573, "Queue in"=w574) -> ("error out"=w576:errorcluster, "Cancel Calibration"=w572:bool)  [unwired: 7 in]
                }
                frame True {
                  n156 = call-dynamic "Check Escala.vi"("error in (no error)"=w588, "Grandeza"=w581, "Multimeter in"=w587) -> ("error out"=w584:errorcluster, "Escala Correta?"=w582:bool, "Multimeter out"=w586:refnum<class "Multimeter.lvclass">)  [unwired: 6 in]
                  n157 = case shown="False" w582 {
                    selector: w582 -> [w591 w598]
                    tunnel: [w592 w599] -> w585
                    tunnel: w584 -> [w594 w599]
                    tunnel: w583 -> [w597 _]
                    tunnel: [w595 w598] -> w580
                    tunnel: w579 -> [w593 _]
                    frame False {
                      n158 = call <vilib>:"Beep.vi"() -> ()  [unwired: 12 in]
                      n159 = Two Button Dialog(message=w597) -> (T button?=w596:bool)  [unwired: 2 in]
                      n160 = Not(x=w596) -> (.not. x?=w590:bool)
                      n161 = call "Cancel Calibration.vi"("error in (no error)"=w594, "Boolean"=w590, "Queue in"=w593) -> ("error out"=w592:errorcluster, "Cancel Calibration"=w589:bool)  [unwired: 7 in]
                      n162 = Or(x=w591, y=w589) -> (x .or. y?=w595:bool)
                    }
                    frame True {
                    }
                  }
                }
              }
            }
          }
          frame True {
          }
        }
      }
      frame "Special Initiate" {
        n163 = Variant To Data(error in=w618, type="", Variant=w613) -> (data=w607:string, error out=w615:errorcluster)
        n164 = case shown="\"34401A\", \"34410A\", \"8846\"" w607 {
          tunnel: w617 -> [w623 w633]
          tunnel: [w623 w627] -> w616
          tunnel: w615 -> [w622 w638]
          tunnel: [w622 w628] -> w614
          tunnel: [w621 w639] -> w612
          tunnel: w611 -> [w621 w639]
          tunnel: w610 -> [w620 w637]
          tunnel: [w620 w636] -> w609
          tunnel: [w619 w624] -> w606
          tunnel: w605 -> [w619 w624]
          frame "False", Default {
          }
          frame "34401A", "34410A", "8846" {
            w634 = "Tensão VDC" ("Grandeza")
            n165 = disable-structure shown="Enabled" {
              disable-tunnel: w638 -> [w646 w647]
              disable-tunnel: w637 -> [w645 w648]
              disable-tunnel: [w644 w648] -> w636
              disable-tunnel: [w641 w647] -> w635
              disable-tunnel: w634 -> [w640 _]
              frame Disabled {
                n166 = call-dynamic "Generate Value.vi"("Grandeza"=w640, "error in (no error)"=w646, "Frequencia"=0.0, "Valor"=0.0, "Calibrator in"=w645) -> ("error out"=w641:errorcluster, "Calibrator out"=w644:refnum<class "Calibrator.lvclass">)  [unwired: 5 in]
              }
              frame Enabled {
              }
            }
            n167 = call-dynamic "Set Measurement.vi"("Escala"=0.1, "error in (no error)"=w635, "Range ON/OFF"=TRUE, "Grandeza Elétrica"=w634, "Multimeter in"=w633) -> ("error out"=w632:errorcluster, "Multimeter out"=w631:refnum<class "Multimeter.lvclass">)  [unwired: 5 in]
            n168 = flat-sequence {
              tunnel: [w651] -> w630
              tunnel: w632 -> [w651]
              tunnel: [w650] -> w629
              tunnel: w631 -> [w650]
              frame #0 {
                n169 = Wait (ms)(milliseconds to wait=u32 1000) -> ()  [unwired: 1 out]
              }
            }
            n170 = call-dynamic "Configure Null.vi"("error in (no error)"=w630, "Multimeter in"=w629) -> ("error out"=w628:errorcluster, "Multimeter out"=w627:refnum<class "Multimeter.lvclass">)  [unwired: 8 in]
          }
        }
      }
      frame "Write to Calibrator" {
        w682 = T8 {"Grandeza"="", "Cel Inicio"="", "Cel Fim"="", "Frequencia"=0.0, "Delay"=0.0, "Valor"=0.0, "Num Medições"=0, "Cel Write"="", "Multiplicador"=0.0, "Message"="", "Escala"=0.0, "Reset"=FALSE}  # Ini File Output
        # "Chama a rotina de medição e \ngravação da planilha o número \nde medições para esse modelo\nde multímetro."
        # "Ajusta o multímetro\npara a medição."
        # "Gera os Valores no Padrão"
        # "Geram os valores no Padrão, configuram os multímetros e o For loop faz a qtde de chamadas para escrever as medições."
        n171 = Variant To Data(error in=w684, type=w682, Variant=w683) -> (data=w670:T8, error out=w681:errorcluster)
        n172 = Unbundle By Name(w670) -> ("Num Medições"=w672:i32, "Grandeza"=w673:string, "Valor"=w679:dbl, "Frequencia"=w678:dbl, "Multiplicador"=w668:dbl, "Escala"=w667:dbl, "Reset"=w657:bool)
        n173 = property on="Bobina" class="Enum (strict)"() -> ("RingText.Text"=w653:string)  [unwired: 2 in, 2 out]
        n174 = Fract/Exp String To Number(string=w653) -> (number=w652:dbl)  [unwired: 3 in, 1 out]
        n175 = case shown="True" w657 {
          tunnel: w681 -> [w685 w690]
          tunnel: w680 -> [w686 w689]
          tunnel: [w685 w688] -> w665
          tunnel: [w686 w687] -> w664
          frame False {
          }
          frame True {
            n176 = call-dynamic "Reset.vi"("error in (no error)"=w690, "Calibrator in"=w689) -> ("error out"=w688:errorcluster, "Calibrator out"=w687:refnum<class "Calibrator.lvclass">)  [unwired: 8 in]
          }
        }
        n177 = call-dynamic "Generate Value.vi"("Multiplicador"=w652, "Grandeza"=w673, "error in (no error)"=w665, "Frequencia"=w678, "Valor"=w679, "Calibrator in"=w664) -> ("error out"=w677:errorcluster, "Calibrator out"=w659:refnum<class "Calibrator.lvclass">)  [unwired: 4 in]
        n178 = Multiply(x=w668, y=w667) -> (x*y=w666:dbl)
        n179 = call-dynamic "Set Measurement.vi"("Escala"=w666, "error in (no error)"=w677, "Range ON/OFF"=TRUE, "Grandeza Elétrica"=w673, "Multimeter in"=w671) -> ("error out"=w676:errorcluster, "Multimeter out"=w663:refnum<class "Multimeter.lvclass">)  [unwired: 5 in]
        n180 = for {
          N: w672 -> [_]
          tunnel: w676 -> [w699]
          tunnel: w675 -> [w702]
          tunnel: [w700] -> w674
          tunnel: w670 -> [w698]
          tunnel: [w694] -> w662
          tunnel: w663 -> [w694]
          tunnel: [w693] -> w660
          tunnel: w661 -> [w693]
          tunnel: [w692] -> w658
          tunnel: w659 -> [w692]
          tunnel: w656 -> [w691]
          tunnel: [w691] -> w655
          i -> [w695]
          n181 = call "Adjust Cell to Write Measurement.vi"("error in (no error)"=w699, "Incremento"=w695, "Ini File Output in"=w698) -> ("error out"=w696:errorcluster, "Ini File Output out"=w697:T8)  [unwired: 7 in]
          n182 = call-poly "Enqueue Message.vi"("Priority Message? (F)"=TRUE, "error in (no error)"=w696, "Message Data"=w697, "Message"="Execute Measurement", "Message Queue"=w702) -> ("error out"=w700:errorcluster)  [unwired: 5 in, 1 out]
        }
      }
      frame "Execute Measurement" {
        w726 = T8 {"Grandeza"="", "Cel Inicio"="", "Cel Fim"="", "Frequencia"=0.0, "Delay"=0.0, "Valor"=0.0, "Num Medições"=0, "Cel Write"="", "Multiplicador"=0.0, "Message"="", "Escala"=0.0, "Reset"=FALSE}  # Ini File Output
        # "Geram os valores no Padrão, configuram os multímetros e o For loop faz a qtde de chamadas para escrever as medições."
        n183 = Variant To Data(error in=w728, type=w726, Variant=w727) -> (data=w725:T8, error out=w711:errorcluster)
        n184 = Unbundle By Name(w725) -> ("Cel Write"=w706:string, "Grandeza"=w705:string, "Delay"=w709:dbl, "Multiplicador"=w708:dbl)
        n185 = call "Time Delay"("error in (no error)"=w711, "Delay Time (s)"=w709) -> ("error out"=w710:errorcluster)  [unwired: 9 in]
        n186 = call-dynamic "Measurement.vi"("error in (no error)"=w710, "Grandeza"=w705, "Multiplicador"=w708, "Multimeter in"=w722) -> ("error out"=w720:errorcluster, "Measurement"=w707:dbl, "Multimeter out"=w721:refnum<class "Multimeter.lvclass">)  [unwired: 5 in]
        n187 = call-poly "Write Data to Cell.vi"("error in"=w720, "Mediçao"=w707, "Cell Name"=w706, "NI_report in"=w724) -> ("error out"=w719:errorcluster, "NI_report out"=w712:refnum<class "NI_report.lvclass">)  [unwired: 6 in]
        n188 = Get Queue Status(queue=w718, error in (no error)=w719) -> (queue out=w713:refnum<queue>, error out=w715:errorcluster, # elements in queue=w716:i32)  [unwired: 1 in, 5 out]
        n189 = Equal To 0?(x=w716) -> (x = 0?=w717:bool)
        n190 = case shown="True" w717 {
          tunnel: w715 -> [w730 w734]
          tunnel: [w730 w733] -> w714
          tunnel: w713 -> [_ w732]
          frame False {
          }
          frame True {
            n191 = call-poly "Enqueue Message.vi"("error in (no error)"=w734, "Message"="Stop", "Message Queue"=w732) -> ("error out"=w733:errorcluster)  [unwired: 7 in, 1 out]
          }
        }
      }
      frame "Open Excel File" {
        # "Error - Display an error dialog. This message is sent by the \"Error Handler\" VIs at the end of other loops in this application."
        n192 = Variant To Data(error in=w753, type=string[] [], Variant=w752) -> (data=w743:string[], error out=w751:errorcluster)
        n193 = Index Array(array=w743) -> (element=w742:string)  [unwired: 1 in]
        n194 = case shown="\"Nova\", Default" "Tipo de Calibração" {
          tunnel: w751 -> [w785 w788]
          tunnel: [w784 w795] -> w735
          tunnel: [w783 w794] -> w748
          tunnel: w742 -> [w782 w789]
          tunnel: [FALSE ("cancelled") w793] -> w738
          frame "Nova", Default {
            n195 = call "Open Excel Template.vi"("error in (no error)"=w785, "Patrimonio"=w782) -> ("error out"=w783:errorcluster, "new path"=w784:path)  [unwired: 8 in]
          }
          frame "Recalibração" {
            n196 = call "FGV Config File.vi"("Error In"=w788, "Set/Get"=enum16{"Get", "Set"}."Get") -> ("Error Out"=w787:errorcluster, "Template File"=w792:path)  [unwired: 7 in, 1 out]
            n197 = Strip Path(path=w792) -> (stripped path=w791:path)  [unwired: 1 out]
            n198 = Build Path(base path=w791, name or relative path=w789) -> (appended path=w790:path)
            n199 = call "File Dialog"("start path"=w790, "error in"=w787) -> ("selected path"=w795:path, "cancelled"=w793:bool, "error out"=w794:errorcluster)  [unwired: 10 in, 1 out]
          }
        }
        n200 = case shown="False" w738 {
          tunnel: [_ w780] -> w750
          tunnel: w735 -> [_ w779]
          tunnel: w748 -> [w760 w778]
          tunnel: w747 -> [w759 w773]
          tunnel: w746 -> [w762 w770]
          tunnel: [w762 w769] -> w745
          tunnel: [w754 w767] -> w744
          tunnel: w740 -> [w761 w766]
          tunnel: [w761 w766] -> w739
          tunnel: w737 -> [w757 w765]
          tunnel: [w756 w765] -> w736
          frame True {
            n201 = Flush Queue(queue=w759, error in (no error)=w760) -> (error out=w755:errorcluster)  [unwired: 2 out]
            n202 = call "UI Config Controls.vi"("Error In"=w755, "UI Configuration"=UI_Config."Initial Config", "UI Data"=w757) -> ("Error Out"=w754:errorcluster, "UI Data 2"=w756:T2)  [unwired: 7 in]
          }
          frame False {
            n203 = call <vilib>:"New Report.vi"("window state (normal)"=T6."maximized", "report type"=T5."Excel", "template (empty)"=w779, "error in (no error)"=w778) -> ("report out"=w780:refnum<class "NI_report.lvclass">, "error out"=w772:errorcluster)  [unwired: 10 in]
            n204 = call-dynamic "Read Model.vi"("error in (no error)"=w772, "Device in"=w770) -> ("error out"=w771:errorcluster, "Model"=w768:string, "Device out"=w769:refnum<class "Multimeter.lvclass">)  [unwired: 7 in]
            n205 = Concatenate Strings("Config Files\\" ("string"), w768, ".ini" ("string")) -> (w774:string)
            n206 = call-poly "Enqueue Message.vi"("error in (no error)"=w771, "Message Data"=w774, "Message"="Read INI File", "Message Queue"=w773) -> ("error out"=w767:errorcluster)  [unwired: 6 in, 1 out]
          }
        }
      }
      frame "Error" {
        # "Error - Display an error dialog. This message is sent by the \"Error Handler\" VIs at the end of other loops in this application."
        n207 = Variant To Data(error in=w806, type=errorcluster {"status"=FALSE, "code"=0, "source"=""} ("error constant"), Variant=w804) -> (data=w802:errorcluster, error out=w801:errorcluster)
        n208 = call <vilib>:"Simple Error Handler.vi"("error in (no error)"=w802) -> ()  [unwired: 4 in, 5 out]
        n209 = Merge Errors(w801) -> (w800:errorcluster)
      }
      frame "Stop" {
        # "Error - Display an error dialog. This message is sent by the \"Error Handler\" VIs at the end of other loops in this application."
        n210 = Flush Queue(queue=w841, error in (no error)=w840) -> (error out=w817:errorcluster)  [unwired: 2 out]
        n211 = call "Data to Excel.vi"("Error In"=w817, "Control"=enum16{"Get", "Set"}."Get") -> ("Error Out"=w836:errorcluster, "Patrim Out"=w831:string, "Controle Out"=w832:string, "Proxima Out"=w837:string, "Hoje out"=w825:string)  [unwired: 5 in]
        n212 = Get Date/Time String(seconds (now)="Próxima Calibração") -> (date string=w835:string)  [unwired: 2 in, 1 out]
        n213 = local read "Número de Controle"() -> (w827:string)
        n214 = local read "Patrimônio"() -> (w826:string)
        n215 = call-poly "Write Data to Cell.vi"("error in"=w836, "Write to Cell"=w835, "Cell Name"=w837, "NI_report in"=w834) -> ("error out"=w829:errorcluster, "NI_report out"=w833:refnum<class "NI_report.lvclass">)  [unwired: 6 in]
        n216 = Get Date/Time String() -> (date string=w823:string)  [unwired: 3 in, 1 out]
        n217 = call-poly "Write Data to Cell.vi"("error in"=w829, "Write to Cell"=w827, "Cell Name"=w832, "NI_report in"=w833) -> ("error out"=w828:errorcluster, "NI_report out"=w830:refnum<class "NI_report.lvclass">)  [unwired: 6 in]
        n218 = call-poly "Write Data to Cell.vi"("error in"=w828, "Write to Cell"=w826, "Cell Name"=w831, "NI_report in"=w830) -> ("error out"=w824:errorcluster, "NI_report out"=w822:refnum<class "NI_report.lvclass">)  [unwired: 6 in]
        n219 = call-poly "Write Data to Cell.vi"("error in"=w824, "Write to Cell"=w823, "Cell Name"=w825, "NI_report in"=w822) -> ("error out"=w821:errorcluster, "NI_report out"=w820:refnum<class "NI_report.lvclass">)  [unwired: 6 in]
        n220 = call-dynamic "Disable Output.vi"("error in (no error)"=w821, "Calibrator in"=w815) -> ("error out"=w816:errorcluster, "Calibrator out"=w814:refnum<class "Calibrator.lvclass">)  [unwired: 8 in]
        n221 = call-dynamic "Reset.vi"("error in (no error)"=w816, "Calibrator in"=w814) -> ("error out"=w812:errorcluster, "Calibrator out"=w813:refnum<class "Calibrator.lvclass">)  [unwired: 8 in]
        n222 = flat-sequence {
          tunnel: [w843] -> w810
          tunnel: w812 -> [w843]
          frame #0 {
            n223 = call <vilib>:"Beep.vi"() -> ()  [unwired: 12 in]
            n224 = One Button Dialog(message="Calibração Finalizada") -> ()  [unwired: 1 in, 1 out]
          }
        }
        n225 = call "UI Config Controls.vi"("Error In"=w810, "UI Configuration"=UI_Config."Initial Config", "UI Data"=w808) -> ("Error Out"=w809:errorcluster, "UI Data 2"=w807:T2)  [unwired: 7 in]
      }
      frame "Confirm Quit" {
        # "Confirm Quit - Message that can confirm whether or not the user wants to exit the application."
        n226 = call-poly "Enqueue Message.vi"("Priority Message? (F)"=TRUE, "error in (no error)"=w854, "Message"="Exit", "Message Queue"=w850) -> ("error out"=w851:errorcluster)  [unwired: 6 in, 1 out]
        n227 = Merge Errors(w851) -> (w852:errorcluster)
      }
      frame "---Copy This Frame---" {
        # "Duplicate this frame when creating new messages.  Change this comment in the duplicated frame to describe this message."
        n228 = Merge Errors(w861) -> (w859:errorcluster)
      }
      frame "Finish Calibration" {
        # "Finishes calibration, close references of instruments, controls and files."
        n229 = Merge Errors(w868) -> (w867:errorcluster)
      }
      frame "Exit" {
        # "Stop the VI"
        # "Release the message queue reference"
        # "Exit - Exit the application."
        n230 = Variant To Data(type=errorcluster {"status"=FALSE, "code"=0, "source"=""} ("error constant"), Variant=w879) -> (data=w880:errorcluster)  [unwired: 1 in, 1 out]
        n231 = call <vilib>:"Simple Error Handler.vi"("error in (no error)"=w880) -> ()  [unwired: 4 in, 5 out]
        n232 = Release Queue(queue=w887, error in (no error)=w882) -> (error out=w873:errorcluster)  [unwired: 1 in, 2 out]
        n233 = call-dynamic "Stop.vi"("error in (no error)"=w873, "Calibrator in"=w872) -> ("error out"=w870:errorcluster, "Calibrator out"=w871:refnum<class "Calibrator.lvclass">)  [unwired: 8 in]
        n234 = call "Close control references.vi"("Error In"=w870, "UI Data"=w878) -> ("Error Out"=w877:errorcluster, "UI Data Out"=w876:T2)  [unwired: 8 in]
        n235 = call "Fire User Event - Stop.vi"("User Event - Stop"=w884) -> ("error out"=w883:errorcluster)  [unwired: 10 in]
        n236 = Merge Errors(w883, w877) -> (w885:errorcluster)
      }
      frame Default {
        # "'Default' case only runs if there is a message that isn't defined in any of the other cases.  Output a programming error."
        n237 = xnode "Error Ring"("parameter 0"=w892) -> ("error out"=w893:errorcluster)
      }
    }
    n238 = call "Error Handler - Message Handling Loop.vi"("error in (no error)"=w24, "Message Queue"=w26) -> ("dup error in"=w25:errorcluster)  [unwired: 8 in, 1 out]
  }
  n239 = while {
    tunnel: w12 -> [w908]
    shift-right: [w906] -> w8
    shift-left: w4 -> [w907]
    tunnel: [w902] -> w5
    stop <- w904 stop-if-true
    # "Event Handling Loop"
    n240 = event shown="[4] \"Multimetro\": Value Change" {
      selector: w907 -> [_ _ _ _ _ _ _]
      dyn-events: [_ _ _ _ _ _ _] -> w906
      timeout: _ -> [_ _ _ _ _ _ _]
      tunnel: [_ _ _ _ _ _ TRUE ("Discard?")] -> w904
      tunnel: w908 -> [w913 w915 w920 w930 w944 w949 w951]
      tunnel: [w912 _ w919 w928 w943 w948 _] -> w905
      tunnel: [w911 w915 w918 w929 w942 w947 w951] -> w903
      event Panel Close? {
        n241 = event-data() -> ()  [unwired: 1 in, 1 out]
        n242 = call-poly "Enqueue Message.vi"("Priority Message? (F)"=TRUE, "Message"="Confirm Quit", "Message Queue"=w913) -> ("error out"=w912:errorcluster, "dup Message Queue"=w911:refnum<queue>)  [unwired: 7 in]
        n243 = event-data("Discard?"=TRUE) -> ()  [unwired: 1 in, 1 out]
      }
      event Application Instance Close {
        n244 = event-data() -> ()  [unwired: 1 in, 1 out]
      }
      event "Finalizar Aplicativo": Value Change {
        n245 = event-data() -> ()  [unwired: 1 in, 1 out]
        n246 = call-poly "Enqueue Message.vi"("Priority Message? (F)"=TRUE, "Message"="Exit", "Message Queue"=w920) -> ("error out"=w919:errorcluster, "dup Message Queue"=w918:refnum<queue>)  [unwired: 7 in]
      }
      event "Iniciar Calibração": Value Change {
        n247 = event-data() -> ()  [unwired: 1 in, 1 out]
        n248 = String Length(string="Patrimônio") -> (length=w927:i32)
        n249 = String Length(string="Número de Controle") -> (length=w926:i32)
        n250 = Equal To 0?(x=w926) -> (x = 0?=w923:bool)
        n251 = Equal To 0?(x=w927) -> (x = 0?=w924:bool)
        n252 = Or(x=w924, y=w923) -> (x .or. y?=w925:bool)
        n253 = case shown="False" w925 {
          tunnel: w930 -> [w937 w939]
          tunnel: [w935 w939] -> w929
          tunnel: [w934 _] -> w928
          tunnel: "Patrimônio" -> [w932 _]
          tunnel: "Número de Controle" -> [w933 _]
          frame False {
            n254 = Build Array(w932, w933) -> (w931:string[])
            n255 = call-poly "Enqueue Message.vi"("Message Data"=w931, "Message"="Pré Configura Calibração", "Message Queue"=w937) -> ("error out"=w934:errorcluster, "dup Message Queue"=w935:refnum<queue>)  [unwired: 7 in]
          }
          frame True {
            n256 = One Button Dialog(message="Preencha Corretetamente os Números\nde Controle e Patrimônio.") -> ()  [unwired: 1 in, 1 out]
          }
        }
      }
      event Value Change {
        n257 = event-data() -> ()  [unwired: 1 in, 1 out]
        n258 = call-poly "Enqueue Message.vi"("Message Data"="Multimetro", "Message"="Config Instrument", "Message Queue"=w944) -> ("error out"=w943:errorcluster, "dup Message Queue"=w942:refnum<queue>)  [unwired: 7 in]
      }
      event "Parar": Value Change {
        n259 = event-data() -> ()  [unwired: 1 in, 1 out]
        n260 = call-poly "Enqueue Message.vi"("Priority Message? (F)"=TRUE, "Message"="Stop", "Message Queue"=w949) -> ("error out"=w948:errorcluster, "dup Message Queue"=w947:refnum<queue>)  [unwired: 7 in]
      }
      event User Event {
        n261 = event-data() -> ()  [unwired: 1 in, 1 out]
      }
    }
    n262 = call "Error Handler - Event Handling Loop.vi"("error in (no error)"=w905, "Message Queue"=w903) -> ("dup error in"=w902:errorcluster)  [unwired: 8 in, 1 out]
  }
  n263 = Unregister For Events(event registration refnum=w8, error in=w5) -> (error out=w9:errorcluster)
  n264 = Merge Errors(w9, w13) -> (w10:errorcluster)
  n265 = call "Destroy User Event - Stop.vi"("error in (no error)"=w10, "User Event - Stop"=w1) -> ("error out"=w6:errorcluster)  [unwired: 9 in]
  n266 = disable-structure shown="Default" {
    disable-tunnel: w6 -> [_ _]
    frame condition #0 (active) {
    }
    frame condition #1 {
      # "Call Quit LabVIEW if running as a built application."
      n267 = Quit LabVIEW(quit? (T)=TRUE) -> ()
    }
  }
